vi "R5DataCollection.vi"(8 "error constant":errorcluster, 10 "Write Once":bool, 11 "LabVIEW Web Service":refnum<class "Web Service.lvclass">) -> (0 "error out":errorcluster={"status"=FALSE, "code"=0, "source"="0"})   [LabVIEW 2016]
uses:
  <vilib>/wsapi/Web Service.lvclass
  <vilib>/Platform/TimedLoop/XDataNode/timing_clust.ctl
  <vilib>/Platform/TimedLoop/XDataNode/nitl_modes.ctl
  <vilib>/Platform/TimedLoop/XDataNode/wakeup.ctl
  <vilib>/Platform/TimedLoop/XDataNode/XDataNode.xnode
  <vilib>/Platform/TimedLoop/XDataNode/XDNodeRunTimeDep.lvlib
  <vilib>/ptbypt/NI_PtbyPt.lvlib
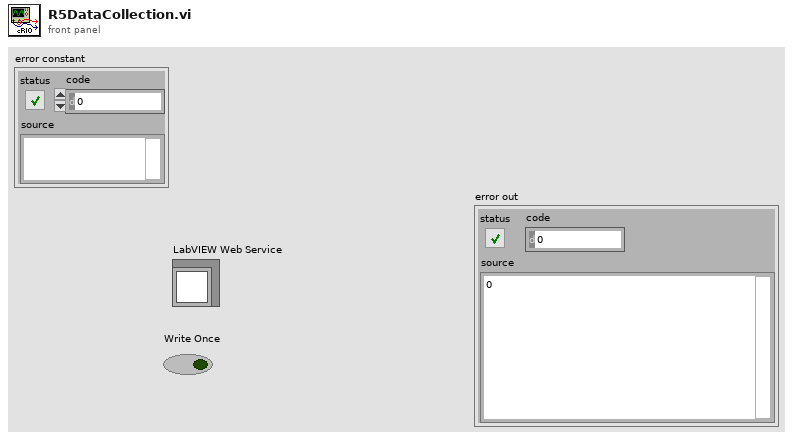
[diagram p1: front panel]
types:
  T1 = typedef "XDNodeRunTimeDep.lvlib/timing_clust.ctl" = cluster{"Expected End [f-1]":u64, "Actual End [f-1]":u64, "Finished Late? [f-1]":bool, "Expected End [i-1]":u64, "Actual End [i-1]":u64, "Finished Late? [i-1]":bool, "Expected Start [i]":u64, "Actual Start [i]":u64, "Expected Start [f]":u64, "Actual Start [f]":u64, "Source Name":string, "Structure Name":string, "Period":i64, "Deadline":i64, "Offset":i64, "Start":i64, "Priority":i32, "Timeout":i32, "Mode":T2, "Wakeup Reason":T3, "Error":errorcluster, "Source Type":string, "Secondary Source Type":string, "Global End Time":u64, "Global Start Time":u64, "Frame Duration":u64, "Iteration Duration":u64, "Assigned CPU":i32, "I/O Scan Engine Mode":u32}
  T2 = typedef "XDNodeRunTimeDep.lvlib/nitl_modes.ctl" = enum32{"No Change", "Process missed periods, maintain original phase", "Discard missed periods, maintain original phase", "Process missed periods, ignore original phase", "Discard missed periods, ignore original phase"}
  T3 = typedef "XDNodeRunTimeDep.lvlib/wakeup.ctl" = enum32{"Normal", "Aborted", "Asynchronous wakeup", "Timing source error", "Timed loop error", "Timeout"}
  T4 = cluster{"Influent Pump":bool, "Effluent Pump":bool}
  T5 = cluster{"Array of Double[0]":dbl, "Array of Double[1]":dbl, "Array of Double[2]":dbl, "Array of Double[3]":dbl, "Array of Double[4]":dbl, "Array of Double[5]":dbl, "Array of Double[6]":dbl, "Array of Double[7]":dbl, "Array of Double[8]":dbl}
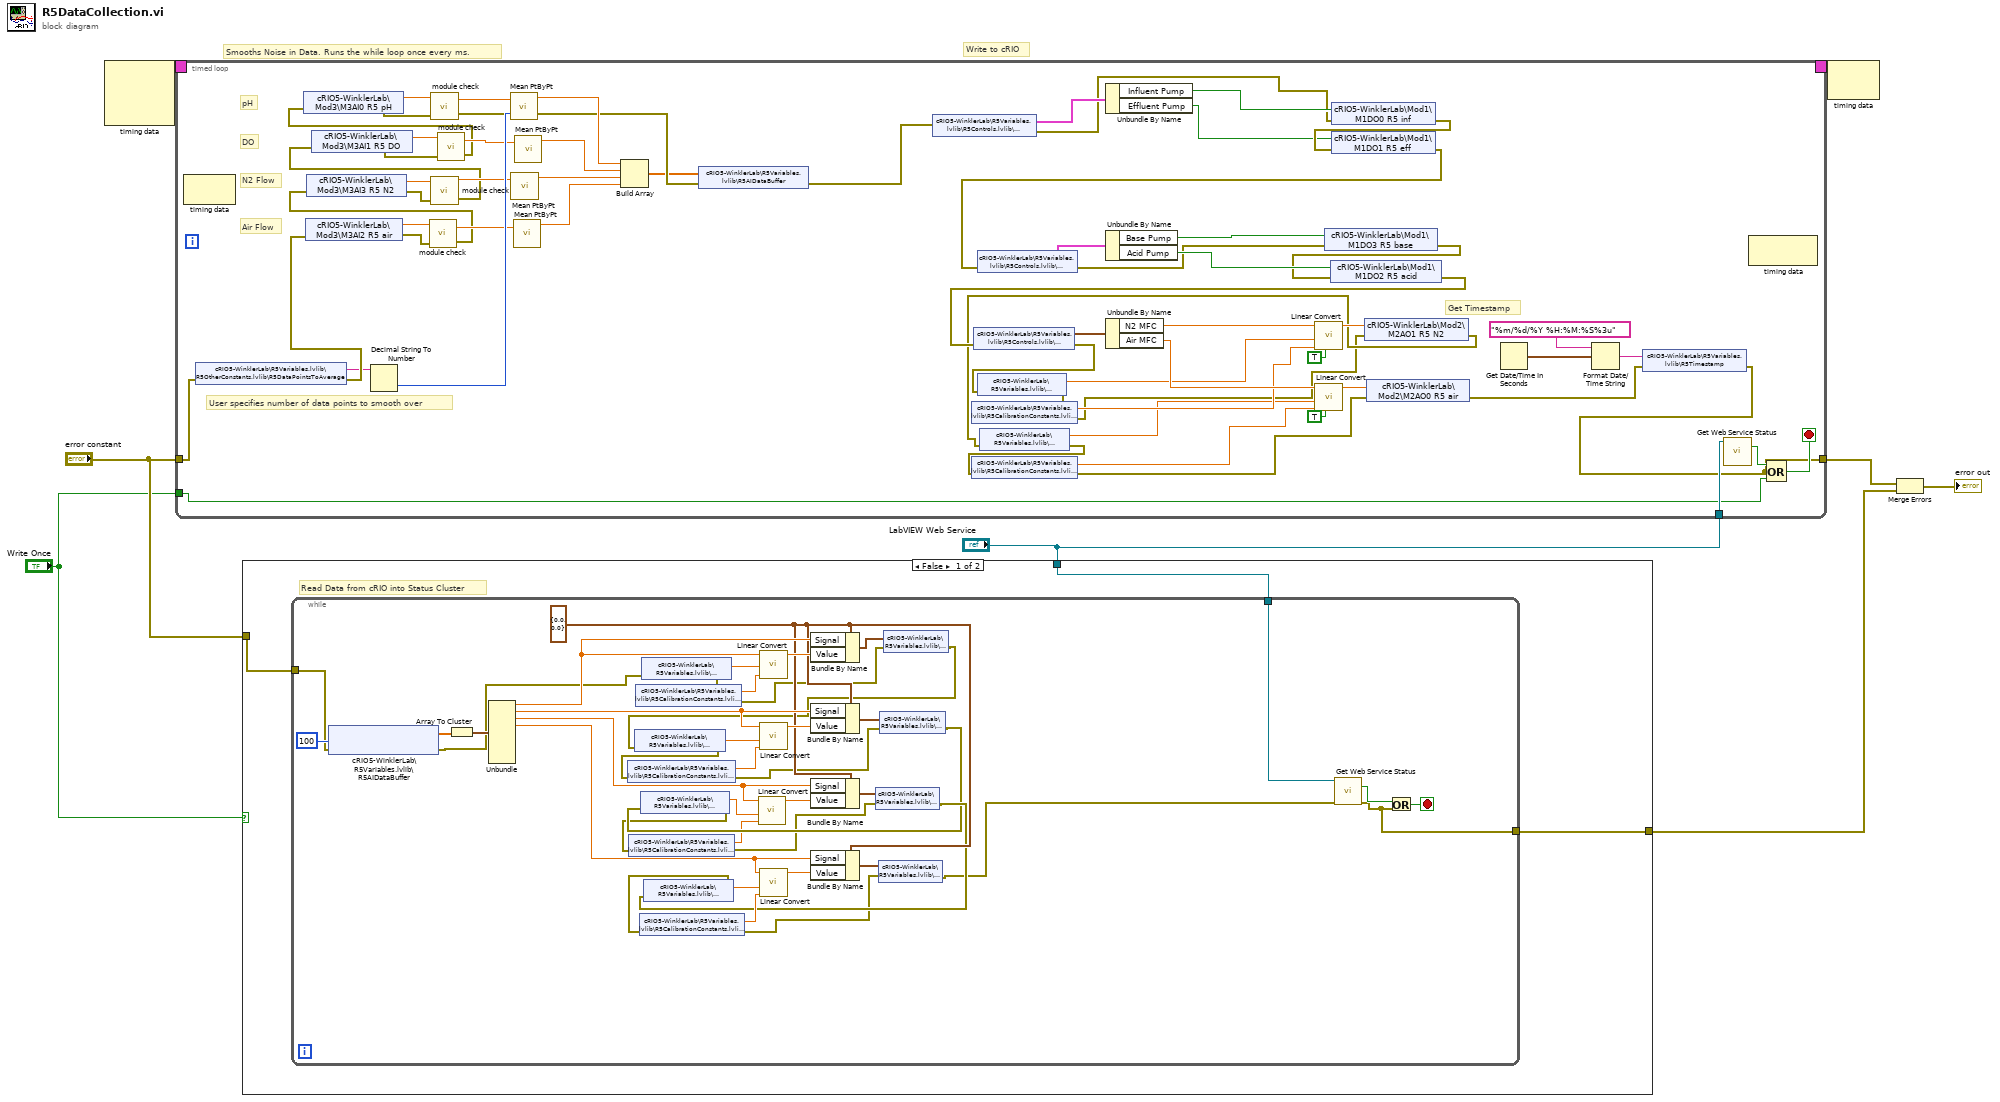
[diagram p0: block diagram]
diagram:
  # "Write to cRIO"
  # "Smooths Noise in Data. Runs the while loop once every ms."
  n1 = node-c288() -> (w8:T1)  [unwired: 3 in]
  n2 = timed-loop {
    timing: w8 -> [_]
    timing-out: [_] -> w7
    tunnel: "error constant" -> [w37]
    tunnel: "LabVIEW Web Service" -> [w70]
    tunnel: "Write Once" -> [w68]
    tunnel: [w25] -> w3
    stop <- w67 stop-if-true
    # "Get Timestamp"
    # "User specifies number of data points to smooth over"
    # "Air Flow"
    # "N2 Flow"
    # "DO"
    # "pH"
    n3 = node-c288() -> ()  [unwired: 1 in, 1 out]
    n4 = shared-variable "cRIO5-WinklerLab\\R5Variables.lvlib\\R5OtherConstants.lvlib\\R5DataPointsToAverage"(error in=w37) -> (w35:string, error out=w36:errorcluster)
    n5 = shared-variable "cRIO5-WinklerLab\\Mod3\\M3AI2 R5 air"(error in=w36) -> (w39:dbl, error out=w38:errorcluster)
    n6 = Decimal String To Number(string=w35) -> (number=w66:i32)  [unwired: 2 in, 1 out]
    n7 = call "module check.vi"("error in"=w38, "Value"=w39) -> ("error constant"=w40:errorcluster, "Value out"=w41:dbl)  [unwired: 1 in]
    n8 = shared-variable "cRIO5-WinklerLab\\Mod3\\M3AI3 R5 N2"(error in=w40) -> (w43:dbl, error out=w42:errorcluster)
    n9 = call "module check.vi"("error in"=w42, "Value"=w43) -> ("error constant"=w44:errorcluster, "Value out"=w45:dbl)  [unwired: 1 in]
    n10 = shared-variable "cRIO5-WinklerLab\\Mod3\\M3AI1 R5 DO"(error in=w44) -> (w47:dbl, error out=w46:errorcluster)
    n11 = call "module check.vi"("error in"=w46, "Value"=w47) -> ("error constant"=w48:errorcluster, "Value out"=w49:dbl)  [unwired: 1 in]
    n12 = shared-variable "cRIO5-WinklerLab\\Mod3\\M3AI0 R5 pH"(error in=w48) -> (w51:dbl, error out=w50:errorcluster)
    n13 = call "module check.vi"("error in"=w50, "Value"=w51) -> ("error constant"=w34:errorcluster, "Value out"=w52:dbl)  [unwired: 1 in]
    n14 = call <vilib>:"Mean PtByPt.vi"("x"=w52, "sample length"=w66) -> ("mean"=w65:dbl)  [unwired: 2 in, 1 out]
    n15 = call <vilib>:"Mean PtByPt.vi"("x"=w45) -> ("mean"=w63:dbl)  [unwired: 3 in, 1 out]
    n16 = call <vilib>:"Mean PtByPt.vi"("x"=w41) -> ("mean"=w64:dbl)  [unwired: 3 in, 1 out]
    n17 = call <vilib>:"Mean PtByPt.vi"("x"=w49) -> ("mean"=w62:dbl)  [unwired: 3 in, 1 out]
    n18 = Build Array(w65, w62, w63, w64) -> (w33:dbl[])
    n19 = shared-variable "cRIO5-WinklerLab\\R5Variables.lvlib\\R5AIDataBuffer"(w33, error in=w34) -> (error out=w32:errorcluster)
    n20 = shared-variable "cRIO5-WinklerLab\\R5Variables.lvlib\\R5Controls.lvlib\\R5SBRManual"(error in=w32) -> (w31:T4, error out=w10:errorcluster)
    n21 = Unbundle By Name(w31) -> ("Influent Pump"=w11:bool, "Effluent Pump"=w12:bool)
    n22 = shared-variable "cRIO5-WinklerLab\\Mod1\\M1DO0 R5 inf"(w11, error in=w10) -> (error out=w58:errorcluster)
    n23 = shared-variable "cRIO5-WinklerLab\\Mod1\\M1DO1 R5 eff"(w12, error in=w58) -> (error out=w9:errorcluster)
    n24 = shared-variable "cRIO5-WinklerLab\\R5Variables.lvlib\\R5Controls.lvlib\\R5pHManual"(error in=w9) -> (w30:cluster{"Acid Pump":bool, "Base Pump":bool}, error out=w29:errorcluster)
    n25 = Unbundle By Name(w30) -> ("Base Pump"=w57:bool, "Acid Pump"=w56:bool)
    n26 = shared-variable "cRIO5-WinklerLab\\Mod1\\M1DO3 R5 base"(w57, error in=w29) -> (error out=w55:errorcluster)
    n27 = shared-variable "cRIO5-WinklerLab\\Mod1\\M1DO2 R5 acid"(w56, error in=w55) -> (error out=w27:errorcluster)
    n28 = shared-variable "cRIO5-WinklerLab\\R5Variables.lvlib\\R5Controls.lvlib\\R5DOManual"(error in=w27) -> (w28:cluster{"Air MFC":dbl, "N2 MFC":dbl}, error out=w15:errorcluster)
    n29 = shared-variable "cRIO5-WinklerLab\\R5Variables.lvlib\\R5CalibrationConstants.lvlib\\R5N2Slope"(error in=w15) -> (w20:dbl, error out=w22:errorcluster)
    n30 = shared-variable "cRIO5-WinklerLab\\R5Variables.lvlib\\R5CalibrationConstants.lvlib\\R5N2Intercept"(error in=w22) -> (w19:dbl, error out=w13:errorcluster)
    n31 = Unbundle By Name(w28) -> ("N2 MFC"=w21:dbl, "Air MFC"=w61:dbl)
    n32 = call "Linear Convert.vi"("Inverse?"=TRUE, "Intercept"=w19, "Slope"=w20, "Signal"=w21) -> ("Result"=w53:dbl)  [unwired: 7 in]
    n33 = shared-variable "cRIO5-WinklerLab\\Mod2\\M2AO1 R5 N2"(w53, error in=w13) -> (error out=w14:errorcluster)
    n34 = shared-variable "cRIO5-WinklerLab\\R5Variables.lvlib\\R5CalibrationConstants.lvlib\\R5AirSlope"(error in=w14) -> (w18:dbl, error out=w23:errorcluster)
    n35 = shared-variable "cRIO5-WinklerLab\\R5Variables.lvlib\\R5CalibrationConstants.lvlib\\R5AirIntercept"(error in=w23) -> (w17:dbl, error out=w16:errorcluster)
    n36 = call "Linear Convert.vi"("Inverse?"=TRUE, "Intercept"=w17, "Slope"=w18, "Signal"=w61) -> ("Result"=w54:dbl)  [unwired: 7 in]
    n37 = shared-variable "cRIO5-WinklerLab\\Mod2\\M2AO0 R5 air"(w54, error in=w16) -> (error out=w24:errorcluster)
    n38 = Get Date/Time In Seconds() -> (seconds since 1Jan1904=w71:timestamp)
    n39 = Format Date/Time String(time format string (%c)="%m/%d/%Y %H:%M:%S%3u", seconds (now)=w71) -> (date/time string=w26:string)  [unwired: 1 in]
    n40 = shared-variable "cRIO5-WinklerLab\\R5Variables.lvlib\\R5Timestamp"(w26, error in=w24) -> (error out=w25:errorcluster)
    n41 = call <vilib>:"Get Web Service Status.vi"("LabVIEW Web Service"=w70) -> ("service stopping?"=w69:bool)  [unwired: 12 in, 2 out]
    n42 = node-c288() -> ()  [unwired: 1 in, 1 out]
    n43 = Compound Arithmetic op=OR(w69, w25, w68) -> (w67:bool)
  }
  n44 = case shown="False" "Write Once" {
    tunnel: "error constant" -> [w77 w120]
    tunnel: "LabVIEW Web Service" -> [w76 _]
    tunnel: [w75 w120] -> w2
    frame False {
      # "Read Data from cRIO into Status Cluster"
      n45 = while {
        tunnel: w77 -> [w81]
        tunnel: [w107] -> w75
        tunnel: w76 -> [w106]
        stop <- w113 stop-if-true
        w108 = cluster{"Signal":dbl, "Value":dbl} {"Signal"=0.0, "Value"=0.0} ("Analog Input")
        n46 = shared-variable "cRIO5-WinklerLab\\R5Variables.lvlib\\R5AIDataBuffer"(error in=w81, u32 100 ("milliseconds to wait")) -> (w82:dbl[], error out=w84:errorcluster)  [unwired: 1 out]
        n47 = Array To Cluster(array=w82) -> (cluster=w119:T5)
        n48 = Unbundle(w119) -> ("Array of Double[0]"=w117:dbl, "Array of Double[1]"=w116:dbl, "Array of Double[2]"=w110:dbl, "Array of Double[3]"=w109:dbl)  [unwired: 5 out]
        n49 = shared-variable "cRIO5-WinklerLab\\R5Variables.lvlib\\R5CalibrationConstants.lvlib\\R5pHSlope"(error in=w84) -> (w105:dbl, error out=w103:errorcluster)
        n50 = shared-variable "cRIO5-WinklerLab\\R5Variables.lvlib\\R5CalibrationConstants.lvlib\\R5pHIntercept"(error in=w103) -> (w104:dbl, error out=w99:errorcluster)
        n51 = call "Linear Convert.vi"("Intercept"=w104, "Slope"=w105, "Signal"=w117) -> ("Result"=w118:dbl)  [unwired: 8 in]
        n52 = Bundle By Name(cluster=w108, "Signal"=w117, "Value"=w118) -> (w98:cluster{"Signal":dbl, "Value":dbl})
        n53 = shared-variable "cRIO5-WinklerLab\\R5Variables.lvlib\\R5Signals.lvlib\\R5pH"(w98, error in=w99) -> (error out=w90:errorcluster)
        n54 = shared-variable "cRIO5-WinklerLab\\R5Variables.lvlib\\R5CalibrationConstants.lvlib\\R5DOSlope"(error in=w90) -> (w91:dbl, error out=w80:errorcluster)
        n55 = shared-variable "cRIO5-WinklerLab\\R5Variables.lvlib\\R5CalibrationConstants.lvlib\\R5DOIntercept"(error in=w80) -> (w79:dbl, error out=w78:errorcluster)
        n56 = call "Linear Convert.vi"("Intercept"=w79, "Slope"=w91, "Signal"=w116) -> ("Result"=w115:dbl)  [unwired: 8 in]
        n57 = Bundle By Name(cluster=w108, "Signal"=w116, "Value"=w115) -> (w97:cluster{"Signal":dbl, "Value":dbl})
        n58 = shared-variable "cRIO5-WinklerLab\\R5Variables.lvlib\\R5Signals.lvlib\\R5DO"(w97, error in=w78) -> (error out=w89:errorcluster)
        n59 = shared-variable "cRIO5-WinklerLab\\R5Variables.lvlib\\R5CalibrationConstants.lvlib\\R5N2Slope"(error in=w89) -> (w88:dbl, error out=w86:errorcluster)
        n60 = shared-variable "cRIO5-WinklerLab\\R5Variables.lvlib\\R5CalibrationConstants.lvlib\\R5N2Intercept"(error in=w86) -> (w85:dbl, error out=w87:errorcluster)
        n61 = call "Linear Convert.vi"("Intercept"=w85, "Slope"=w88, "Signal"=w110) -> ("Result"=w111:dbl)  [unwired: 8 in]
        n62 = Bundle By Name(cluster=w108, "Signal"=w110, "Value"=w111) -> (w96:cluster{"Signal":dbl, "Value":dbl})
        n63 = shared-variable "cRIO5-WinklerLab\\R5Variables.lvlib\\R5Signals.lvlib\\R5N2"(w96, error in=w87) -> (error out=w95:errorcluster)
        n64 = shared-variable "cRIO5-WinklerLab\\R5Variables.lvlib\\R5CalibrationConstants.lvlib\\R5AirSlope"(error in=w95) -> (w102:dbl, error out=w100:errorcluster)
        n65 = shared-variable "cRIO5-WinklerLab\\R5Variables.lvlib\\R5CalibrationConstants.lvlib\\R5AirIntercept"(error in=w100) -> (w101:dbl, error out=w93:errorcluster)
        n66 = call "Linear Convert.vi"("Intercept"=w101, "Slope"=w102, "Signal"=w109) -> ("Result"=w112:dbl)  [unwired: 8 in]
        n67 = Bundle By Name(cluster=w108, "Signal"=w109, "Value"=w112) -> (w94:cluster{"Signal":dbl, "Value":dbl})
        n68 = shared-variable "cRIO5-WinklerLab\\R5Variables.lvlib\\R5Signals.lvlib\\R5Air"(w94, error in=w93) -> (error out=w92:errorcluster)
        n69 = call <vilib>:"Get Web Service Status.vi"("LabVIEW Web Service"=w106, "error in (no error)"=w92) -> ("service stopping?"=w114:bool, "error out"=w107:errorcluster)  [unwired: 11 in, 1 out]
        n70 = Or(x=w114, y=w107) -> (x .or. y?=w113:bool)
      }
    }
    frame True {
    }
  }
  n71 = node-c288(w7) -> ()  [unwired: 1 out]
  n72 = Merge Errors(w3, w2) -> (→"error out":errorcluster)
